vi "Bayer 3X3 Buffer.vi"(7 "Bayer Array":u8[][](array[numeric]), 8 "Col Inde":i32, 9 "Row Index":i32, 10 "Height":i32, 11 "Width":i32) -> (3 "3X3 Buffer":T1)   [LabVIEW 2017]
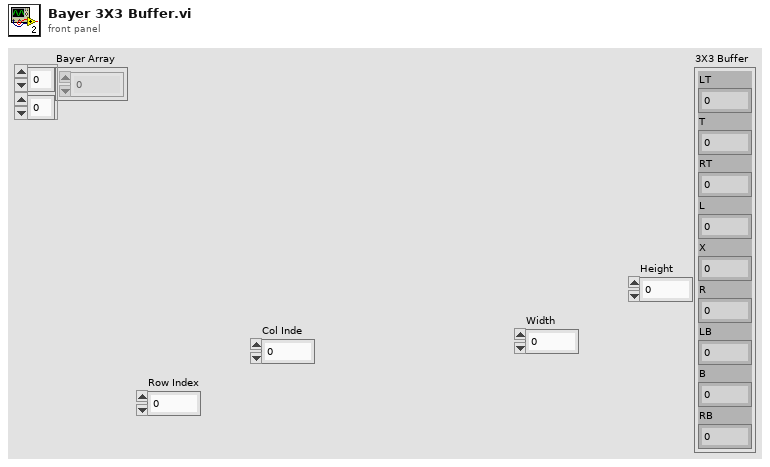
[diagram p1: front panel]
types:
  T1 = cluster{"LT":u16, "T":u16, "RT":u16, "L":u16, "X":u16, "R":u16, "LB":u16, "B":u16, "RB":u16}
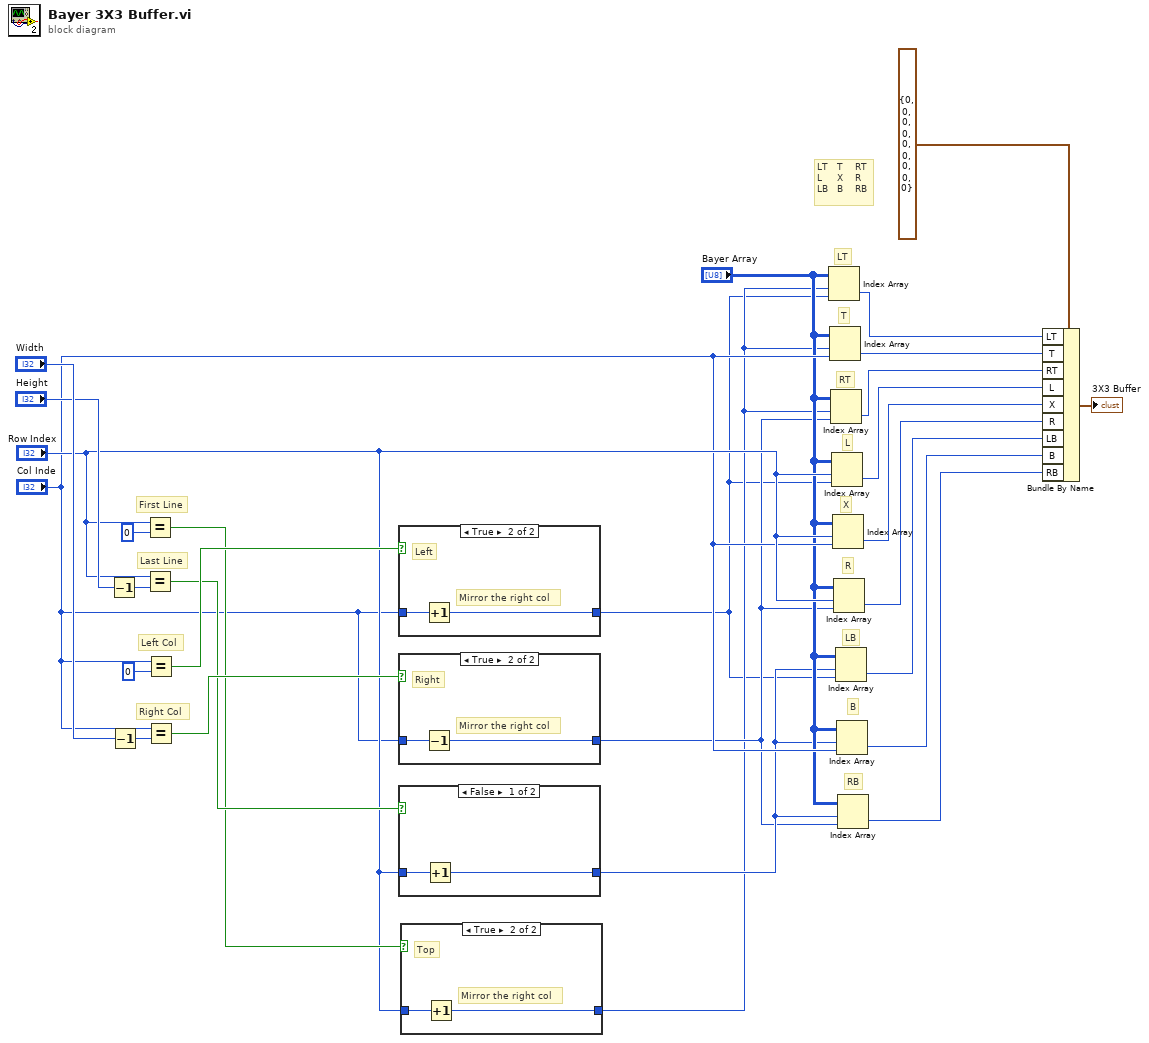
[diagram p0: block diagram]
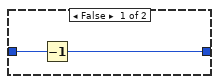
[diagram p2: hidden frame]
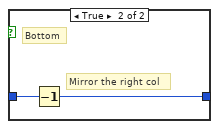
[diagram p3: hidden frame]
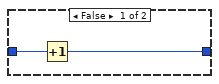
[diagram p4: hidden frame]
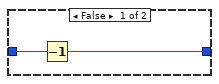
[diagram p5: hidden frame]
diagram:
  # "RB"
  # "B"
  # "LB"
  # "R"
  # "X"
  # "L"
  # "RT"
  # "T"
  # "LT"
  # "LT   T    RT\nL     X    R\nLB   B    RB"
  # "Right Col"
  # "Left Col"
  # "Last Line"
  # "First Line"
  n1 = Decrement(x="Height") -> (x-1=w27:i32)
  n2 = Decrement(x="Width") -> (x-1=w25:i32)
  n3 = Equal?(x="Row Index", y=0) -> (x = y?=w19:bool)
  n4 = Equal?(x="Row Index", y=w27) -> (x = y?=w20:bool)
  n5 = Equal?(x="Col Inde", y=0) -> (x = y?=w22:bool)
  n6 = Equal?(x="Col Inde", y=w25) -> (x = y?=w21:bool)
  n7 = case shown="True" w22 {
    tunnel: "Col Inde" -> [w30 w32]
    tunnel: [w29 w31] -> w2
    frame False {
      n8 = Decrement(x=w30) -> (x-1=w29:i32)
    }
    frame True {
      # "Mirror the right col"
      # "Left"
      n9 = Increment(x=w32) -> (x+1=w31:i32)
    }
  }
  n10 = case shown="True" w21 {
    tunnel: "Col Inde" -> [w34 w36]
    tunnel: [w33 w35] -> w14
    frame False {
      n11 = Increment(x=w34) -> (x+1=w33:i32)
    }
    frame True {
      # "Mirror the right col"
      # "Right"
      n12 = Decrement(x=w36) -> (x-1=w35:i32)
    }
  }
  n13 = case shown="False" w20 {
    tunnel: "Row Index" -> [w38 w40]
    tunnel: [w37 w39] -> w15
    frame False {
      n14 = Increment(x=w38) -> (x+1=w37:i32)
    }
    frame True {
      # "Mirror the right col"
      # "Bottom"
      n15 = Decrement(x=w40) -> (x-1=w39:i32)
    }
  }
  n16 = case shown="True" w19 {
    tunnel: "Row Index" -> [w42 w44]
    tunnel: [w41 w43] -> w3
    frame False {
      n17 = Decrement(x=w42) -> (x-1=w41:i32)
    }
    frame True {
      # "Mirror the right col"
      # "Top"
      n18 = Increment(x=w44) -> (x+1=w43:i32)
    }
  }
  n19 = Index Array(array="Bayer Array", index (row)=w3, index (col)=w2) -> (element=w12:u8)
  n20 = Index Array(array="Bayer Array", index (row)=w3, index (col)="Col Inde") -> (element=w11:u8)
  n21 = Index Array(array="Bayer Array", index (row)=w3, index (col)=w14) -> (element=w10:u8)
  n22 = Index Array(array="Bayer Array", index (row)="Row Index", index (col)=w2) -> (element=w9:u8)
  n23 = Index Array(array="Bayer Array", index (row)="Row Index", index (col)="Col Inde") -> (element=w8:u8)
  n24 = Index Array(array="Bayer Array", index (row)="Row Index", index (col)=w14) -> (element=w7:u8)
  n25 = Index Array(array="Bayer Array", index (row)=w15, index (col)=w2) -> (element=w6:u8)
  n26 = Index Array(array="Bayer Array", index (row)=w15, index (col)="Col Inde") -> (element=w5:u8)
  n27 = Index Array(array="Bayer Array", index (row)=w15, index (col)=w14) -> (element=w4:u8)
  n28 = Bundle By Name(cluster=T1 {"LT"=0, "T"=0, "RT"=0, "L"=0, "X"=0, "R"=0, "LB"=0, "B"=0, "RB"=0} ("input cluster"), "LT"=w12, "T"=w11, "RT"=w10, "L"=w9, "X"=w8, "R"=w7, "LB"=w6, "B"=w5, "RB"=w4) -> (→"3X3 Buffer":T1)
